vi "SR430.get discriminator slope.vi"(0 "i ref in":refnum<vi>, 5 "error in (no error)":errorcluster) -> (14 "i ref out":refnum<vi>, 16 "discriminator slope (rising)":bool, 19 "error out":errorcluster)   [LabVIEW 2014, in "SR430.lvlib"]
doc: "gets the discriminator slope from the BaseProcess.i attribute"
uses:
  SR430.lvlib
  CS_Core/BaseProcess/BaseProcess.lvlib
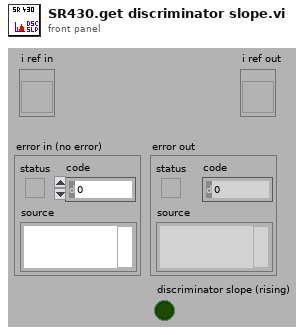
[diagram p1: front panel]
types:
  T1 = typedef "BaseProcess.lvlib/BaseProcess.i attribute.ctl" = cluster{"EventStatus":string, "EventError":i32, "PresetEvtWatchD":i32, "PresetPdcWatchD":i32, "EventTimeout":i32, "PeriodicInterval":i32, "Interface":string[], "Address":string[], "Special":string[], "PeriodicError":i32, "PeriodicStatus":string, "SuperProc":string, "Descriptors":T2[], "CaseRef":refnum<vi>, "PdcRef":refnum<vi>, "Thread Ref":refnum<vi>, "eventErrorID":i32, "eventStatusID":i32, "periodicErrorID":i32, "periodicStatusID":i32, "pdcCtrID":i32}
  T2 = typedef "BaseProcess.lvlib/BaseProcess.descriptor definition.ctl" = cluster{"selector":string, "descriptor":T3}
  T3 = typedef "BaseProcess.lvlib/BaseProcess.descriptor string definition.ctl" = string
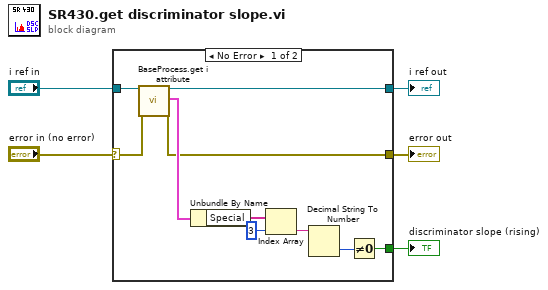
[diagram p0: block diagram]
diagram:
  n1 = case shown="No Error" "error in (no error)" {
    selector: "error in (no error)" -> [w6 w16]
    tunnel: "i ref in" -> [w15 w17]
    tunnel: [w13 w17] -> w4
    tunnel: [w12 w16] -> w3
    tunnel: [w7 _] -> w2
    frame No Error {
      n2 = call "BaseProcess.get i attribute.vi"("i ref in"=w15, "error in (no error)"=w6) -> ("i ref out"=w13:refnum<vi>, "i attribute"=w14:T1, "error out"=w12:errorcluster)  [unwired: 15 in]
      n3 = Unbundle By Name(w14) -> ("Special"=w11:string[])
      n4 = Index Array(array=w11, index=3 ("Index")) -> (element=w9:string)
      n5 = Decimal String To Number(string=w9) -> (number=w8:i32)  [unwired: 2 in, 1 out]
      n6 = Not Equal To 0?(x=w8) -> (x != 0?=w7:bool)
    }
    frame Error {
    }
  }
  "error out" <- w3
  "i ref out" <- w4
  "discriminator slope (rising)" <- w2
